vi "HGF_GPG.appendData2Variant.vi"(0 "initData":variant, 1 "password":string, 2 "key-id":string, 3 "GPG-folder":path, 4 "create keypair":bool, 5 "error in (no error)":errorcluster, 6 "keyring":path, 7 "Sec keyring":path, 8 "options file":path, 9 "Trust DB":path, 11 "Language":bool) -> (14 "dup initData":variant, 19 "error out":errorcluster)   [LabVIEW 2012, in "HGF_GPG.lvlib" / "HGF_GPG.lvclass"]
uses:
  HGF_GPG.lvclass
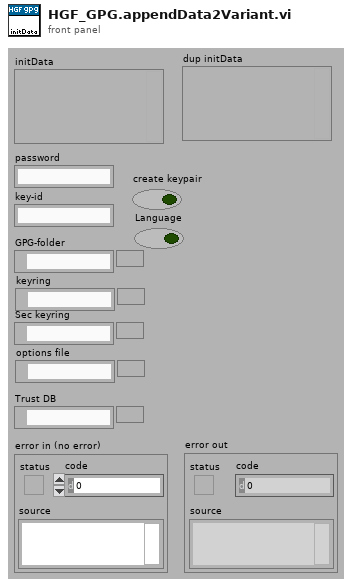
[diagram p1: front panel]
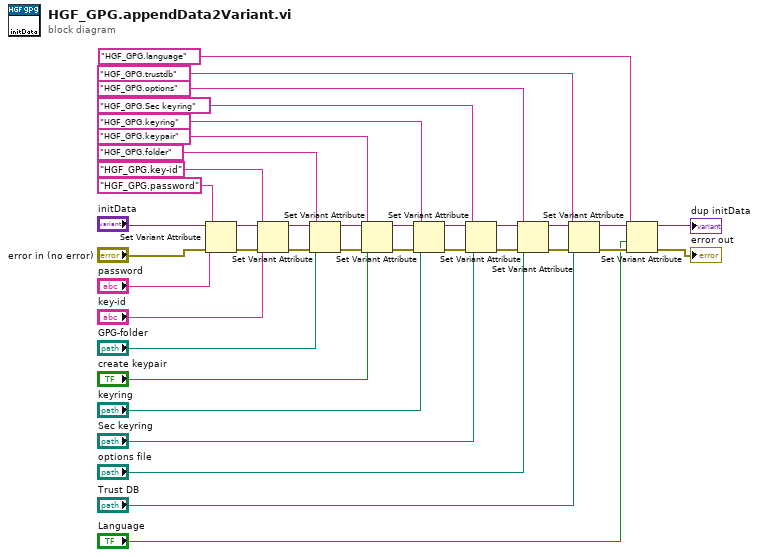
[diagram p0: block diagram]
diagram:
  n1 = Set Variant Attribute(Variant="initData", name="HGF_GPG.password", value="password", error in="error in (no error)") -> (Variant out=w37:variant, error out=w35:errorcluster)  [unwired: 1 out]
  n2 = Set Variant Attribute(Variant=w37, name="HGF_GPG.key-id", value="key-id", error in=w35) -> (Variant out=w30:variant, error out=w29:errorcluster)  [unwired: 1 out]
  n3 = Set Variant Attribute(Variant=w30, name="HGF_GPG.folder", value="GPG-folder", error in=w29) -> (Variant out=w26:variant, error out=w25:errorcluster)  [unwired: 1 out]
  n4 = Set Variant Attribute(Variant=w26, name="HGF_GPG.keypair", value="create keypair", error in=w25) -> (Variant out=w21:variant, error out=w22:errorcluster)  [unwired: 1 out]
  n5 = Set Variant Attribute(Variant=w21, name="HGF_GPG.keyring", value="keyring", error in=w22) -> (Variant out=w15:variant, error out=w16:errorcluster)  [unwired: 1 out]
  n6 = Set Variant Attribute(Variant=w15, name="HGF_GPG.Sec keyring", value="Sec keyring", error in=w16) -> (Variant out=w14:variant, error out=w13:errorcluster)  [unwired: 1 out]
  n7 = Set Variant Attribute(Variant=w14, name="HGF_GPG.options", value="options file", error in=w13) -> (Variant out=w10:variant, error out=w9:errorcluster)  [unwired: 1 out]
  n8 = Set Variant Attribute(Variant=w10, name="HGF_GPG.trustdb", value="Trust DB", error in=w9) -> (Variant out=w6:variant, error out=w4:errorcluster)  [unwired: 1 out]
  n9 = Set Variant Attribute(Variant=w6, name="HGF_GPG.language", value="Language", error in=w4) -> (Variant out=→"dup initData":variant, error out=→"error out":errorcluster)  [unwired: 1 out]
